vi "Read Meta Value.vi"(8 "error in (no error)":errorcluster, 10 "Meta Name":string, 11 "Config Element in":refnum<class "Config Element.lvclass">) -> (0 "error out":errorcluster, 2 "Meta Value":string, 3 "Config Element out":refnum<class "Config Element.lvclass">)   [LabVIEW 2020, in "CDM-Config.lvlib" / "Config Element.lvclass"]
doc: "Looks up and returns the value for a single meta field. If the meta name does not exist an error is returned."
uses:
  Config Element.lvclass
  Config Element.lvclass/Config Element.ctl
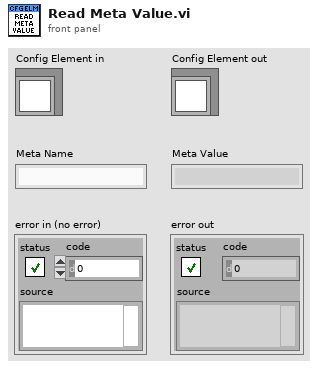
[diagram p1: front panel]
types:
  T1 = typedef "CDM-Config.lvlib/Config Element.lvclass/Ref Data.ctl" = cluster{"Node Info":T2, "Owner":refnum<class>, "Changed":bool, "Name":string, "Value":string, "Meta Data":T3[]}
  T2 = typedef "CDM-Config.lvlib/Node Info.ctl" = cluster{"Index":i32, "Parent":i32, "Children":i32[]}
  T3 = typedef "CDM-Config.lvlib/Meta Data.ctl" = cluster{"Name":string, "Value":string}
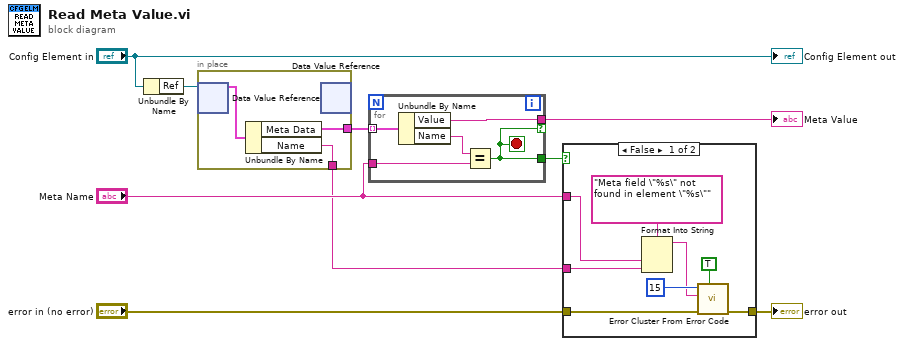
[diagram p0: block diagram]
diagram:
  n1 = Unbundle By Name("Config Element in") -> ("Ref"=w9:refnum<data-value>)
  n2 = in-place {
    in-place-border: [w11] -> w7
    in-place-border: [w10] -> w1
    n3 = in-place-dvr #1(w9) -> (w12:T1)  [unwired: 1 out]
    n4 = Unbundle By Name(w12) -> ("Meta Data"=w11:T3[], "Name"=w10:string)
    n5 = in-place-dvr #1() -> ()  [unwired: 1 in, 2 out]
  }
  n6 = for {
    tunnel: w7 -> [w17] mode=indexing
    tunnel: "Meta Name" -> [w15]
    tunnel: [w14] -> w3 if=w13
    tunnel: [w13] -> w6
    stop <- w13 stop-if-true
    n7 = Unbundle By Name(w17) -> ("Value"=w14:string, "Name"=w16:string)
    n8 = Equal?(x=w16, y=w15) -> (x = y?=w13:bool)
  }
  "Meta Value" <- w3
  n9 = case shown="False" w6 {
    tunnel: "error in (no error)" -> [w23 w26]
    tunnel: [w19 w26] -> w4
    tunnel: "Meta Name" -> [w24 _]
    tunnel: w1 -> [w18 _]
    frame False {
      n10 = Format Into String(format string="Meta field \"%s\" not found in element \"%s\"", w24, w18) -> (resulting string=w20:string)  [unwired: 2 in, 1 out]
      n11 = call <vilib>:"Error Cluster From Error Code.vi"("show call chain? (False)"=TRUE, "error in (no error)"=w23, "error message (\"\")"=w20, "error code (0)"=15) -> ("error out"=w19:errorcluster)  [unwired: 5 in]
    }
    frame True {
    }
  }
  "error out" <- w4
  "Config Element out" <- "Config Element in"
